vi "Write Ctls.vi"(10 "Ctls":T1, 11 "Cooler UI in":refnum<class "Live User Controller.lvclass">) -> (3 "Cooler UI out":refnum<class "Live User Controller.lvclass">)   [LabVIEW 2018, in "Live User Controller.lvclass"]
doc: "Write the control refnums from the user interface into the actor object."
uses:
  Live User Controller.lvclass
  ControlRefs.ctl
  Live User Controller.lvclass/Live User Controller.ctl
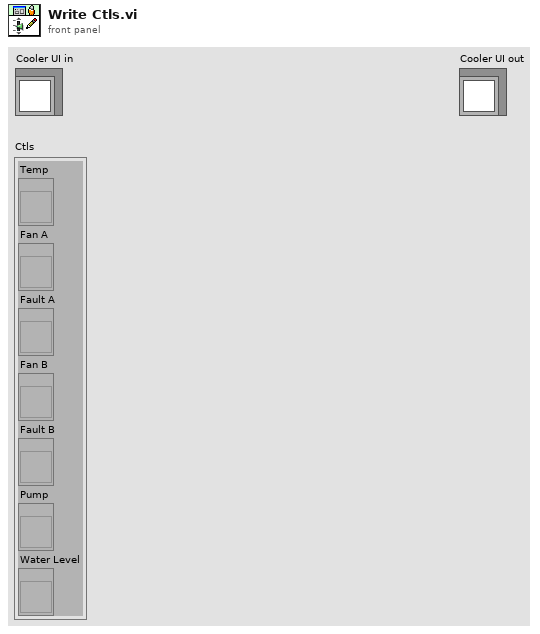
[diagram p1: front panel]
types:
  T1 = typedef "Live User Controller.lvclass/ControlRefs.ctl" = cluster{"Temp":refnum<vi>, "Fan A":refnum<vi>, "Fault A":refnum<vi>, "Fan B":refnum<vi>, "Fault B":refnum<vi>, "Pump":refnum<vi>, "Water Level":refnum<vi>}
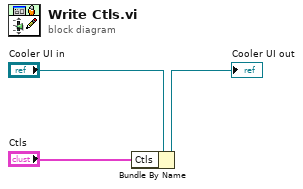
[diagram p0: block diagram]
diagram:
  n1 = Bundle By Name(cluster="Cooler UI in", "Ctls"="Ctls") -> (→"Cooler UI out":refnum<class "Live User Controller.lvclass">)
